vi "ProdaNG.FreeData.vi"(8 "error in (no error)":errorcluster, 10 "Pointers":u32) -> (0 "error out":errorcluster)   [LabVIEW 2016]
doc: "This function releases the memory of Arrays, which is allocated by the DLL. \nParameter:\narrayOfPtrs is an Array pointer that has been filled by DLL functions, which pass back result lists. After calling this function, the content of this parameter is invalid and must not be used any further on."
uses:
  prodllNG.dll
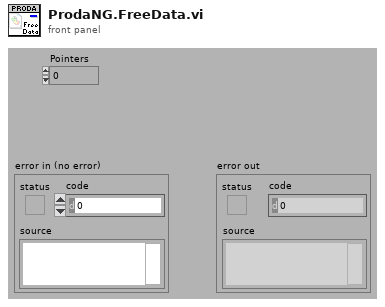
[diagram p1: front panel]
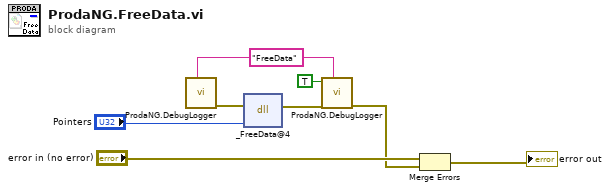
[diagram p0: block diagram]
diagram:
  w7 = "FreeData" ("cmd")
  n1 = call "ProdaNG.DebugLogger.vi"("cmd"=w7) -> ("error out"=w4:errorcluster)  [unwired: 10 in]
  n2 = dll-call lib="D:/Maszup/WABCO/SVN/LineTraceSystem/SOFTWARE/sources/Database/ProdaNG/prodllNG.dll" fn="_FreeData@4" ("ProDll.dll:InitProDll")(error in=w4, "data"="Pointers") -> (error out=w5:errorcluster)  [unwired: 4 in, 1 out]
  n3 = call "ProdaNG.DebugLogger.vi"("cmd"=w7, "error in (no error)"=w5, "done? (F)"=TRUE) -> ("error out"=w1:errorcluster)  [unwired: 8 in]
  n4 = Merge Errors("error in (no error)", w1) -> (→"error out":errorcluster)
